vi "Check If Pixels Belong In Sector.vi"() -> (3 "FIFO Timeout?":bool)   [LabVIEW 2013]
uses:
  Single Sector Pixel Cluster.ctl
  Globals/Sector Parameter Global.vi
  Globals/Pixel Location Global.vi
  <vilib>/rvi/FIFO/Fifo_Resource/nirvififoEmulationReadFpgaImpl.vi
  <vilib>/rvi/DataTransferAndStorage/Container/Common/niFpgaContainerGetUniqueNameForEmu.vi
  <vilib>/rvi/FIFO/Fifo_Resource/nirvififoEmulationWriteFpgaImpl.vi
  <vilib>/rvi/DataTransferAndStorage/Container/XNode/niFpgaContainer.xnode
  <vilib>/rvi/FIFO/Fifo_Resource/nirvififoEmulationRead.vi
  <vilib>/rvi/FIFO/Fifo_Resource/nirvififoEmulationWrite.vi
  FPGA Image Processing.lvlib
panel:
  out "End of  Data?":bool
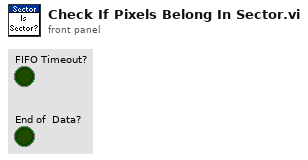
[diagram p1: front panel]
types:
  T1 = typedef "Sector Parameter Cluster.ctl" = cluster{"Start Angle":fxp<+,17,3>, "End Angle":fxp<+,17,3>, "Inner Radius":u16, "Outter Radius":u16, "Hinge X":u16, "Hinge Y":u16, "NumWingSectors":u8}
  T2 = typedef "Single Sector Pixel Cluster.ctl" = cluster{"Sector #":u8, "Pixel Value":u8}
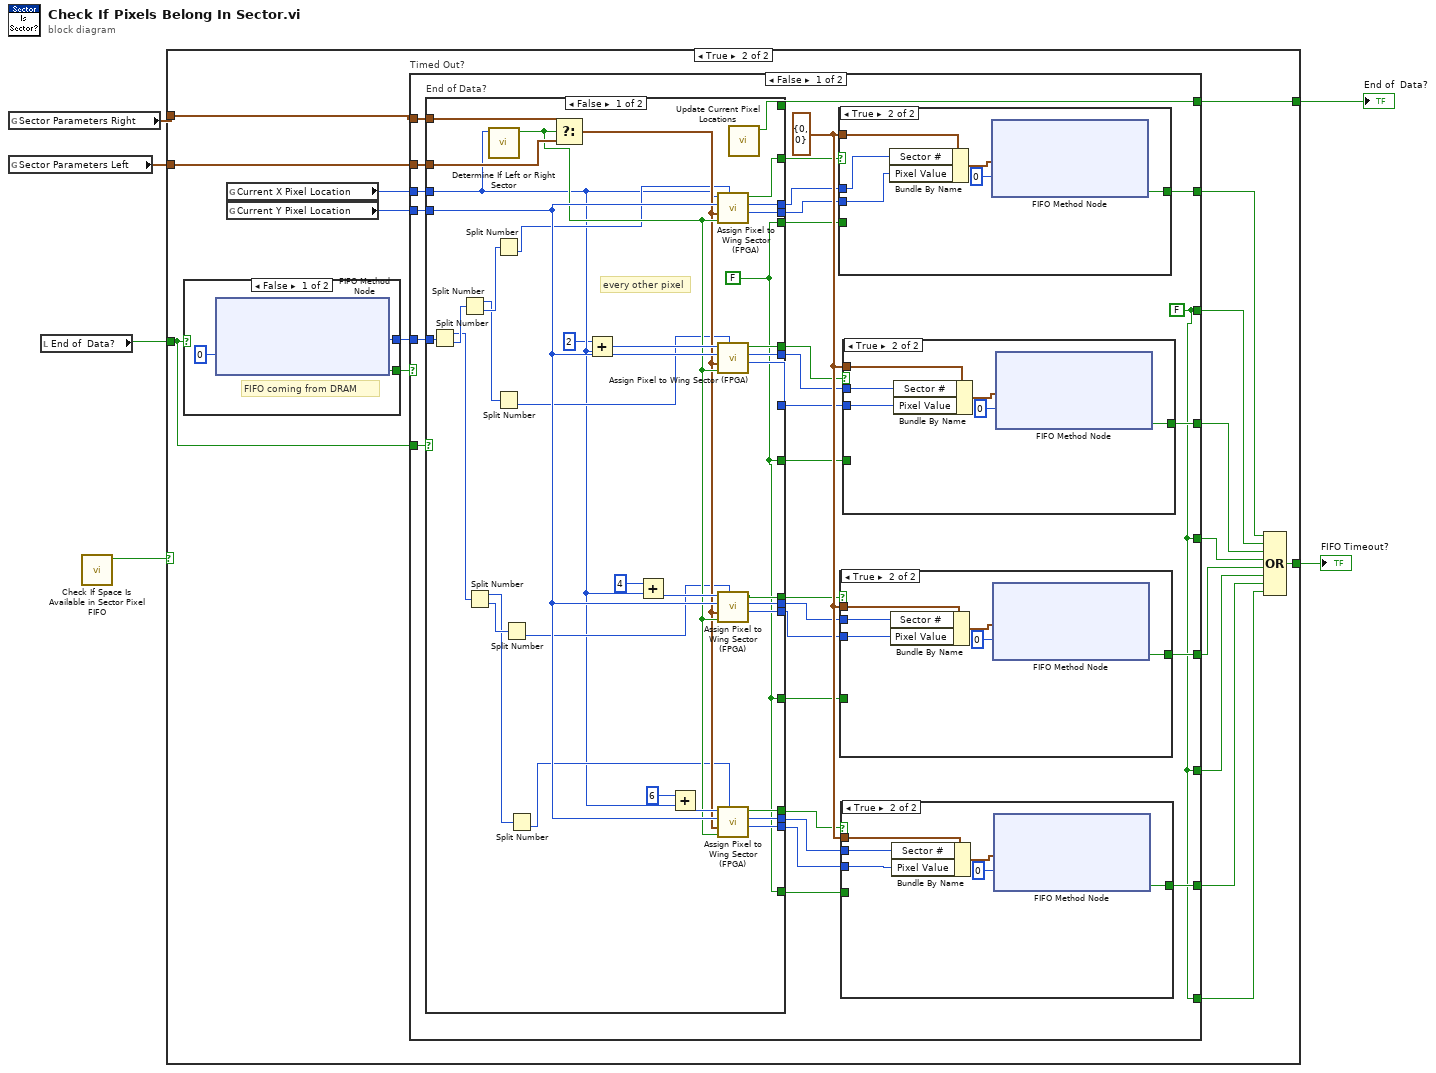
[diagram p0: block diagram]
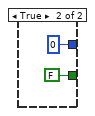
[diagram p3: hidden frame]
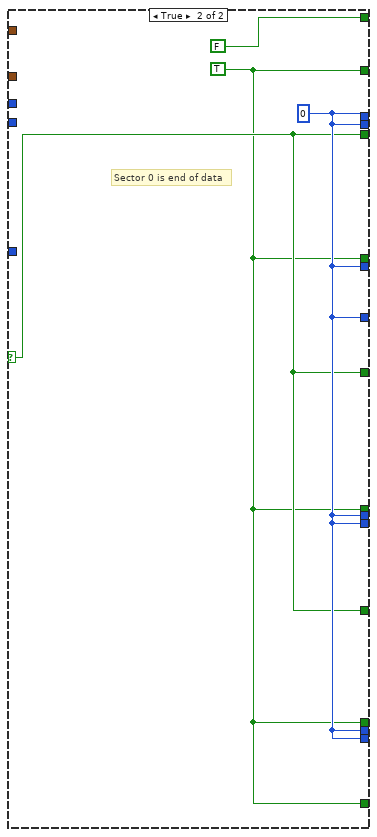
[diagram p4: hidden frame]
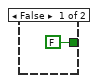
[diagram p5: hidden frame]
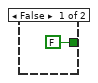
[diagram p6: hidden frame]
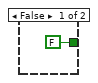
[diagram p7: hidden frame]
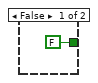
[diagram p8: hidden frame]
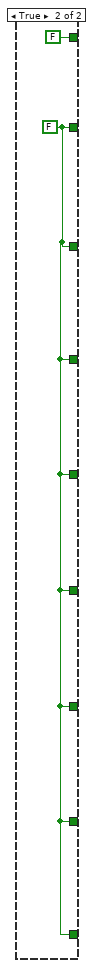
[diagram p9: hidden frame]
diagram:
  n1 = global read "Sector Parameter Global.vi" "Sector Parameters Right"() -> (w2:T1)
  n2 = global read "Sector Parameter Global.vi" "Sector Parameters Left"() -> (w1:T1)
  n3 = local read "End of  Data?"() -> (w4:bool)
  n4 = call "Check If Space Is Available in Sector Pixel FIFO.vi"() -> ("Space Avaliable?"=w3:bool)  [unwired: 11 in]
  n5 = case shown="True" w3 {
    tunnel: [_ w12] -> w5
    tunnel: [w7 w11] -> w6
    tunnel: w4 -> [w7 w10]
    tunnel: w2 -> [_ w9]
    tunnel: w1 -> [_ w8]
    frame False {
    }
    frame True {
      n6 = case shown="False" w10 {
        tunnel: [w26 FALSE ("Timed Out?")] -> w24
        tunnel: [w25 u64 0 ("Element")] -> w21
        frame False {
          # "FIFO coming from DRAM"
          n7 = xnode ("FIFO Method Node")("Timeout"=0) -> ("Element"=w25:u64, "Timed Out?"=w26:bool)  [unwired: 1 in, 1 out]
        }
        frame True {
        }
      }
      n8 = global read "Pixel Location Global.vi" "Current X Pixel Location"() -> (w23:u16)
      n9 = global read "Pixel Location Global.vi" "Current Y Pixel Location"() -> (w22:u16)
      n10 = case "Timed Out?" shown="False" w24 {
        tunnel: w23 -> [w49 _]
        tunnel: w22 -> [w58 _]
        tunnel: w21 -> [w56 _]
        tunnel: [w57 w129] -> w20
        tunnel: [w34 w129] -> w19
        tunnel: [w55 w129] -> w18
        tunnel: [w34 w129] -> w17
        tunnel: [w54 w129] -> w16
        tunnel: [w34 w129] -> w15
        tunnel: [w52 w129] -> w14
        tunnel: [w34 w129] -> w13
        tunnel: w9 -> [w51 _]
        tunnel: w8 -> [w50 _]
        tunnel: [w36 FALSE ("End of Average Data?")] -> w11
        tunnel: w10 -> [w35 _]
        frame False {
          w34 = FALSE ("Timed Out?")
          w53 = T2 {"Sector #"=0, "Pixel Value"=0} ("Single Sector Pixel")
          n11 = case "End of Data?" shown="False" w35 {
            selector: w35 -> [_ w97]
            tunnel: w58 -> [w92 _]
            tunnel: w56 -> [w88 _]
            tunnel: w51 -> [w84 _]
            tunnel: w50 -> [w83 _]
            tunnel: w49 -> [w63 _]
            tunnel: [w79 w96] -> w48
            tunnel: [w78 w98] -> w47
            tunnel: [w77 w98] -> w46
            tunnel: [w76 w96] -> w45
            tunnel: [w75 w98] -> w44
            tunnel: [w73 w98] -> w43
            tunnel: [w72 w96] -> w42
            tunnel: [w71 w98] -> w41
            tunnel: [w69 w98] -> w40
            tunnel: [w68 w96] -> w39
            tunnel: [w67 w98] -> w38
            tunnel: [w66 w98] -> w37
            tunnel: [w64 FALSE ("End of data?")] -> w36
            tunnel: [w62 w97] -> w33
            tunnel: [w62 w97] -> w32
            tunnel: [w62 w97] -> w31
            tunnel: [w62 w96] -> w30
            frame False {
              w62 = FALSE
              # "every other pixel"
              n12 = Split Number(x=w88) -> (hi(x)=w90:u32, lo(x)=w91:u32)
              n13 = Split Number(x=w91) -> (hi(x)=w87:u16, lo(x)=w89:u16)
              n14 = Split Number(x=w90) -> (hi(x)=w85:u16, lo(x)=w86:u16)
              n15 = call "Determine If Left or Right Sector.vi"("X Pixel Location"=w63) -> ("Right Sector?"=w82:bool)  [unwired: 10 in]
              n16 = Split Number(x=w89) -> (lo(x)=w80:u8)  [unwired: 1 out]
              n17 = Split Number(x=w87) -> (lo(x)=w74:u8)  [unwired: 1 out]
              n18 = Split Number(x=w86) -> (lo(x)=w70:u8)  [unwired: 1 out]
              n19 = Split Number(x=w85) -> (lo(x)=w65:u8)  [unwired: 1 out]
              n20 = Select(t=w84, s=w82, f=w83) -> (s? t:f=w81:T1)
              n21 = Add(x=u16 2, y=w63) -> (x+y=w95:u16)
              n22 = Add(x=u16 4, y=w63) -> (x+y=w94:u16)
              n23 = Add(x=u16 6, y=w63) -> (x+y=w93:u16)
              n24 = call "Assign Pixel to Wing Sector (FPGA).vi"("Pixel Intensity In"=w80, "Right Wing?"=w82, "Sector Parameters"=w81, "Pixel Y"=w92, "Pixel X"=w63) -> ("Pixel Intensity Out"=w77:u8, "sector #"=w78:u8, "output valid"=w79:bool)  [unwired: 1 in, 2 out]
              n25 = call "Assign Pixel to Wing Sector (FPGA).vi"("Pixel Intensity In"=w74, "Right Wing?"=w82, "Sector Parameters"=w81, "Pixel Y"=w92, "Pixel X"=w95) -> ("Pixel Intensity Out"=w73:u8, "sector #"=w75:u8, "output valid"=w76:bool)  [unwired: 1 in, 2 out]
              n26 = call "Assign Pixel to Wing Sector (FPGA).vi"("Pixel Intensity In"=w70, "Right Wing?"=w82, "Sector Parameters"=w81, "Pixel Y"=w92, "Pixel X"=w94) -> ("Pixel Intensity Out"=w69:u8, "sector #"=w71:u8, "output valid"=w72:bool)  [unwired: 1 in, 2 out]
              n27 = call "Assign Pixel to Wing Sector (FPGA).vi"("Pixel Intensity In"=w65, "Right Wing?"=w82, "Sector Parameters"=w81, "Pixel Y"=w92, "Pixel X"=w93) -> ("Pixel Intensity Out"=w66:u8, "sector #"=w67:u8, "output valid"=w68:bool)  [unwired: 1 in, 2 out]
              n28 = call "Update Current Pixel Locations.vi"() -> ("End of data?"=w64:bool)  [unwired: 11 in]
            }
            frame True {
              w98 = u8 0 ("sector #")
              w96 = TRUE ("output valid")
              # "Sector 0 is end of data"
            }
          }
          n29 = case shown="True" w48 {
            tunnel: w53 -> [_ w127]
            tunnel: [FALSE ("Timed Out?") w124] -> w57
            tunnel: w47 -> [_ w122]
            tunnel: w46 -> [_ w123]
            tunnel: w33 -> [_ _]
            frame False {
            }
            frame True {
              n30 = Bundle By Name(cluster=w127, "Sector #"=w122, "Pixel Value"=w123) -> (w125:T2)
              n31 = xnode ("FIFO Method Node")("Element"=w125, "Timeout"=0) -> ("Timed Out?"=w124:bool)  [unwired: 1 in, 1 out]
            }
          }
          n32 = case shown="True" w42 {
            tunnel: w53 -> [_ w113]
            tunnel: [FALSE ("Timed Out?") w110] -> w54
            tunnel: w41 -> [_ w108]
            tunnel: w40 -> [_ w109]
            tunnel: w31 -> [_ _]
            frame False {
            }
            frame True {
              n33 = Bundle By Name(cluster=w113, "Sector #"=w108, "Pixel Value"=w109) -> (w111:T2)
              n34 = xnode ("FIFO Method Node")("Element"=w111, "Timeout"=0) -> ("Timed Out?"=w110:bool)  [unwired: 1 in, 1 out]
            }
          }
          n35 = case shown="True" w39 {
            tunnel: w53 -> [_ w106]
            tunnel: [FALSE ("Timed Out?") w103] -> w52
            tunnel: w38 -> [_ w101]
            tunnel: w37 -> [_ w102]
            tunnel: w30 -> [_ _]
            frame False {
            }
            frame True {
              n36 = Bundle By Name(cluster=w106, "Sector #"=w101, "Pixel Value"=w102) -> (w104:T2)
              n37 = xnode ("FIFO Method Node")("Element"=w104, "Timeout"=0) -> ("Timed Out?"=w103:bool)  [unwired: 1 in, 1 out]
            }
          }
          n38 = case shown="True" w45 {
            tunnel: w53 -> [_ w120]
            tunnel: [FALSE ("Timed Out?") w117] -> w55
            tunnel: w44 -> [_ w115]
            tunnel: w43 -> [_ w116]
            tunnel: w32 -> [_ _]
            frame False {
            }
            frame True {
              n39 = Bundle By Name(cluster=w120, "Sector #"=w115, "Pixel Value"=w116) -> (w118:T2)
              n40 = xnode ("FIFO Method Node")("Element"=w118, "Timeout"=0) -> ("Timed Out?"=w117:bool)  [unwired: 1 in, 1 out]
            }
          }
        }
        frame True {
          w129 = FALSE ("Timed Out?")
        }
      }
      n41 = Compound Arithmetic op=OR(w20, w19, w18, w17, w16, w15, w14, w13) -> (w12:bool)
    }
  }
  "End of  Data?" <- w6
  "FIFO Timeout?" <- w5
